vi "Boolean_ErrorMessageContainsString.vi"() -> ()   [LabVIEW 2017, in "Assertion.Tests.lvlib" / "AssertIsNotBoolean.lvlib"]
uses:
  AssertIsNotBoolean.lvlib
  Assertion/Assertion.lvlib
panel:
  out "error out":errorcluster
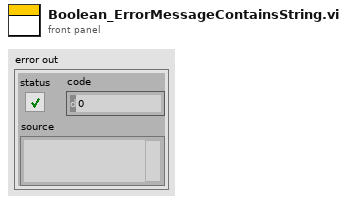
[diagram p1: front panel]
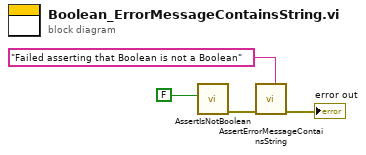
[diagram p0: block diagram]
diagram:
  n1 = call "AssertIsNotBoolean.vi"("Actual"=FALSE) -> ("error out"=w3:errorcluster)  [unwired: 10 in]
  n2 = call "AssertErrorMessageContainsString.vi"("Expected"="Failed asserting that Boolean is not a Boolean", "error in (no error)"=w3) -> ("error out"=→"error out":errorcluster)  [unwired: 9 in]
